vi "Path Edit.vi"() -> ()   [LabVIEW 2013]
uses:
  Global Variables.vi
panel:
  in  "Index":i32=8
  in  "Direction":u16(ring) items=["Forward", "Backward"]
  in  "Enabled":bool=TRUE
  in  "Voltage Schedule":u16(ring) items=["Constant", "Ramp", "Fn. Generator", "Formula"]
  in  "Apply to All":bool
  in  "Fill Orientation":u16(ring) items=["Horizontal", "Vertical"]
  in  "Smooth Segments":dbl=12.0
  in  "Speed Schedule":u16(ring) items=["Constant", "Ramp", "Fn. Generator", "Formula"]
  in  "Speed (µm/s)":dbl=8.0
  in  "Voltage (V)":dbl=8.0
  in  "Speed Settings":bool
  in  "Voltage Settings":bool
  in  "Fill Spacing":dbl=0.1
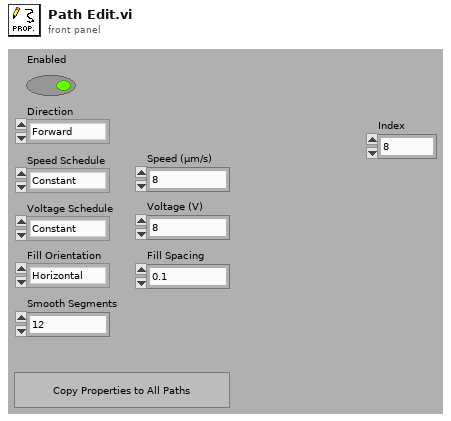
[diagram p1: front panel]
types:
  T1 = enum32{"invalid app kind", "Development System", "Run Time System", "Student Edition", "Embedded LabVIEW", "Evaluation", "Custom"}
  T2 = enum32{"Invalid", "Standard", "Closed", "Hidden", "Minimized", "Maximized"}
  T3 = cluster{"Enabled":bool, "Direction":u16, "Fill Orientation":u16, "Smooth Segments":dbl, "Fill Spacing":dbl, "Speed (µm/s)":cluster{"Schedule":u16, "Value":dbl, "Start Value":dbl, "End Value":dbl, "Min Value":dbl, "Max Value":dbl, "Duty Cycle (%)":dbl, "Signal Type":u16, "Cycle Number":dbl, "Phase (degrees)":dbl}, "Voltage (V)":cluster{"Schedule":u16, "Value":dbl, "Start Value":dbl, "End Value":dbl, "Min Value":dbl, "Max Value":dbl, "Duty Cycle (%)":dbl, "Signal Type":u16, "Cycle Number":dbl, "Phase (degrees)":dbl}}[]
  T4 = cluster{"Enabled":bool, "Direction":u16, "Fill Orientation":u16, "Smooth Segments":dbl, "Fill Spacing":dbl, "Speed (µm/s)":cluster{"Schedule":u16, "Value":dbl, "Start Value":dbl, "End Value":dbl, "Min Value":dbl, "Max Value":dbl, "Duty Cycle (%)":dbl, "Signal Type":u16, "Cycle Number":dbl, "Phase (degrees)":dbl}, "Voltage (V)":cluster{"Schedule":u16, "Value":dbl, "Start Value":dbl, "End Value":dbl, "Min Value":dbl, "Max Value":dbl, "Duty Cycle (%)":dbl, "Signal Type":u16, "Cycle Number":dbl, "Phase (degrees)":dbl}}
  T5 = cluster{"Schedule":u16, "Value":dbl, "Start Value":dbl, "End Value":dbl, "Min Value":dbl, "Max Value":dbl, "Duty Cycle (%)":dbl, "Signal Type":u16, "Cycle Number":dbl, "Phase (degrees)":dbl}
  T6 = cluster{"Schedule":u16, "Value":dbl, "Start Value":dbl, "End Value":dbl, "Min Value":dbl, "Max Value":dbl, "Duty Cycle (%)":dbl, "Speed Signal Type":u16, "Cycle Number":dbl, "Phase (degrees)":dbl}
  T7 = cluster{"Core":cluster{"Current VI Reference":refnum<vi>, "Close Panel on Exit?":bool}}
  T8 = cluster{"Current VI Reference":refnum<vi>, "Close Panel on Exit?":bool}
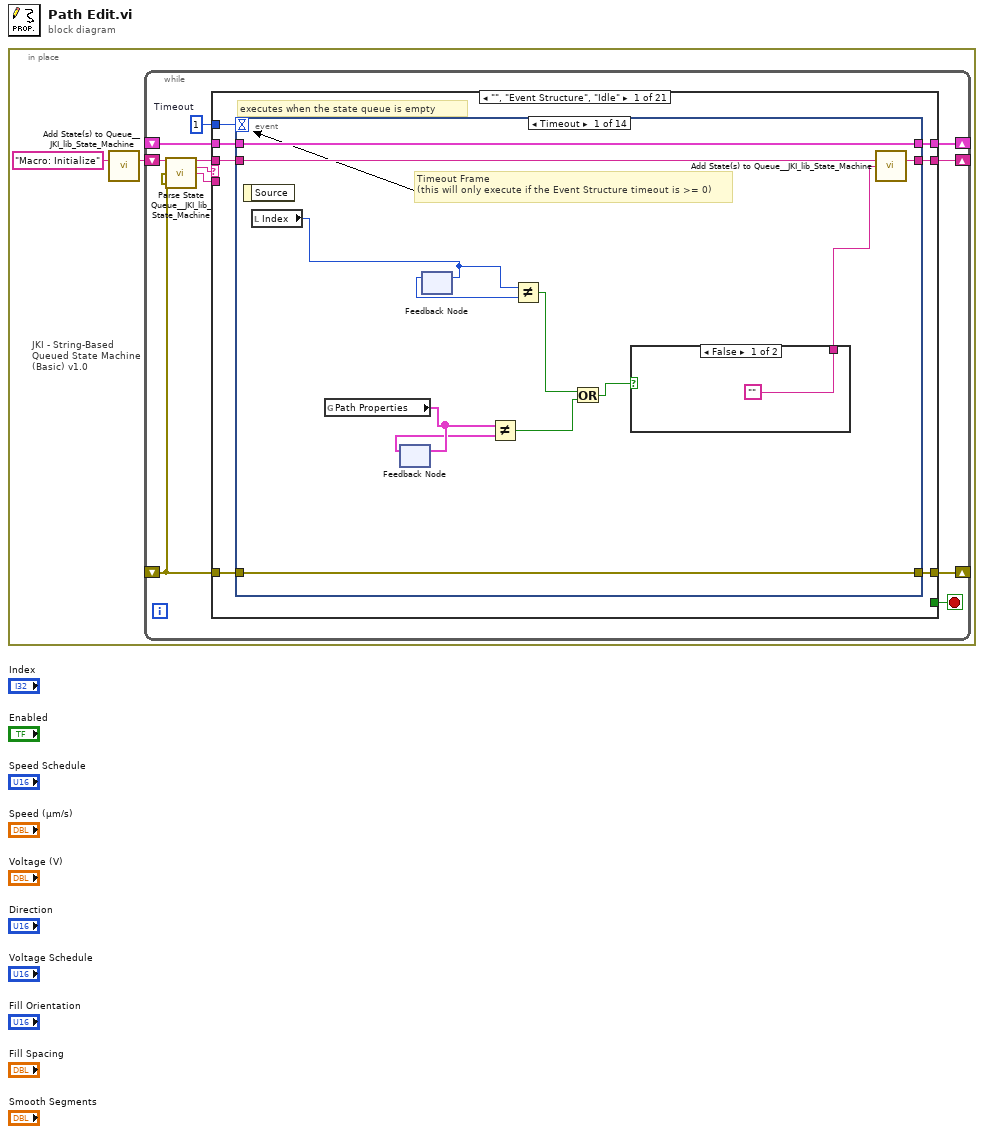
[diagram p0: block diagram]
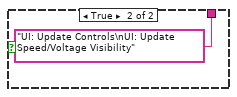
[diagram p2: hidden frame]
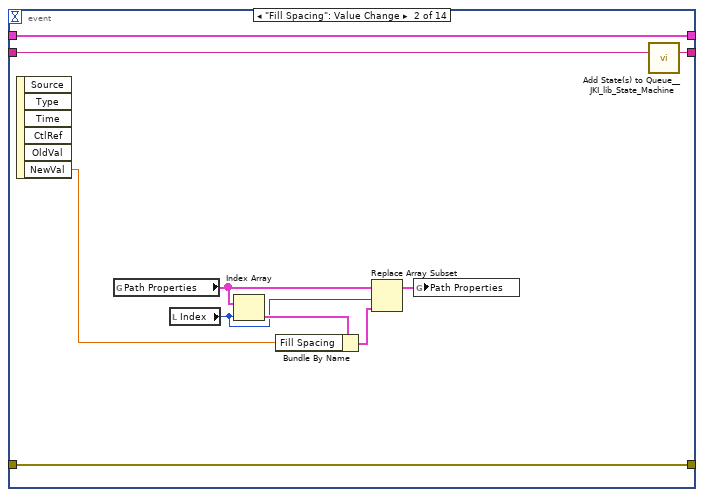
[diagram p3: hidden frame]
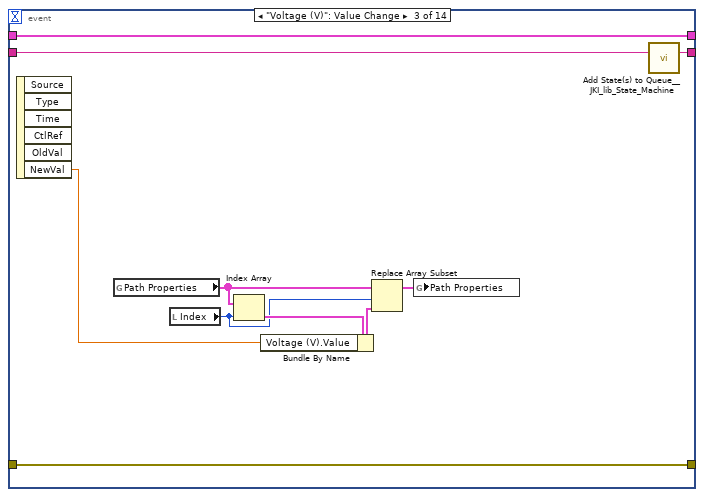
[diagram p4: hidden frame]
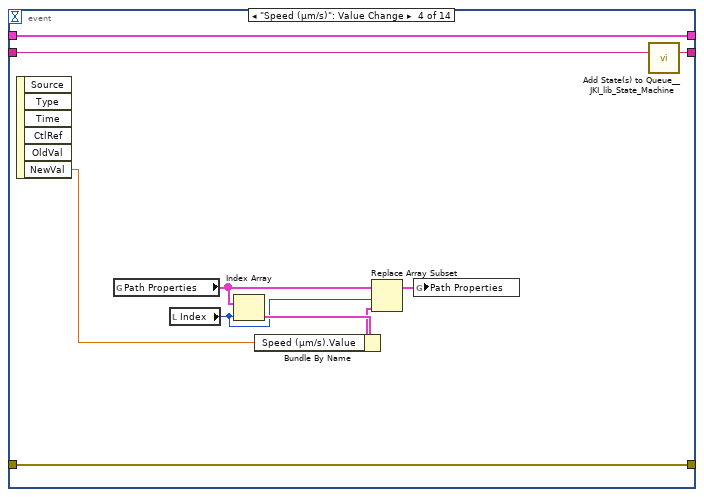
[diagram p5: hidden frame]
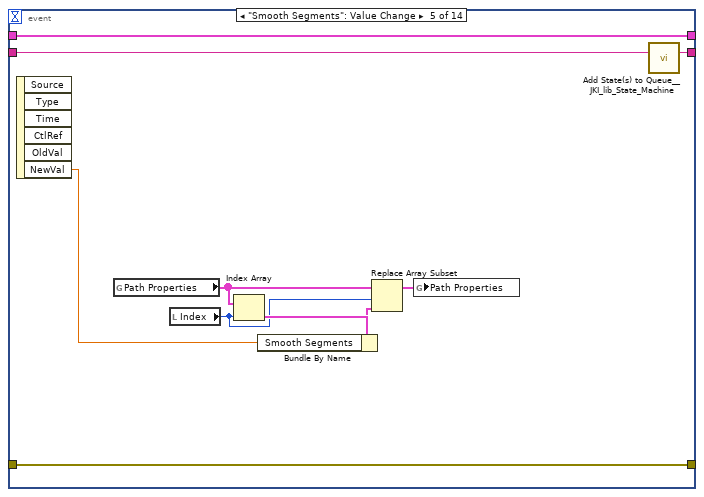
[diagram p6: hidden frame]
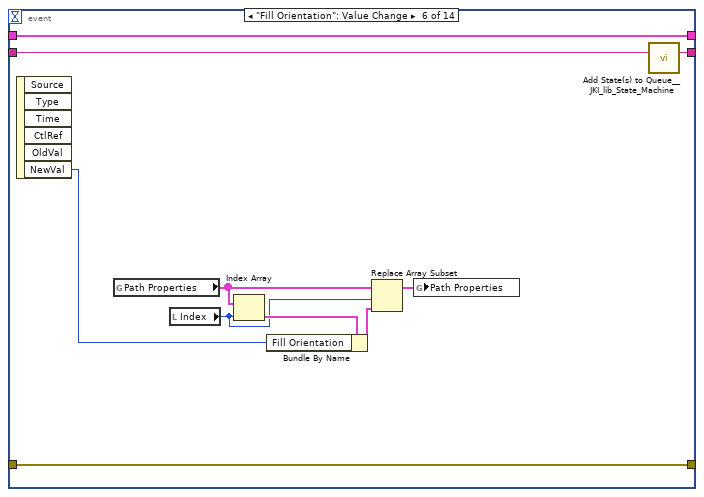
[diagram p7: hidden frame]
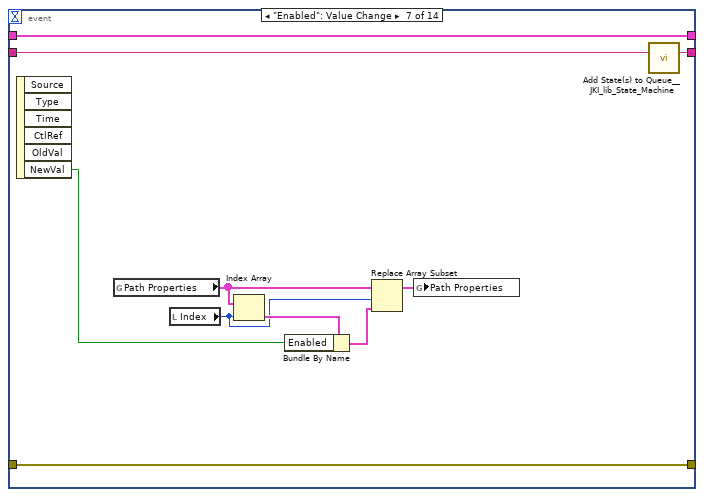
[diagram p8: hidden frame]
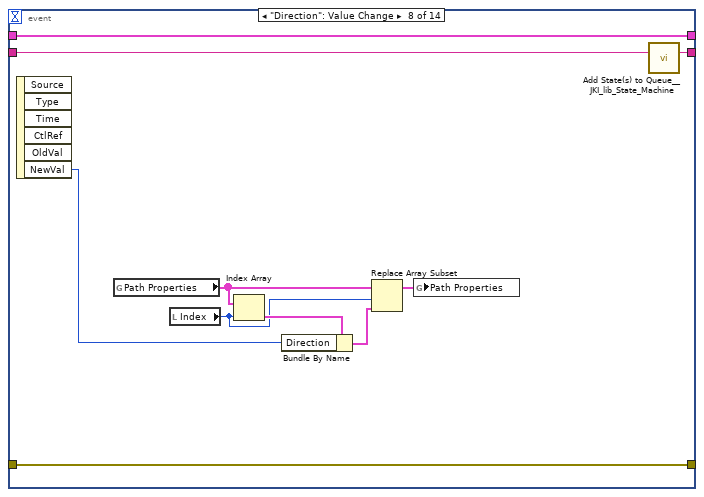
[diagram p9: hidden frame]
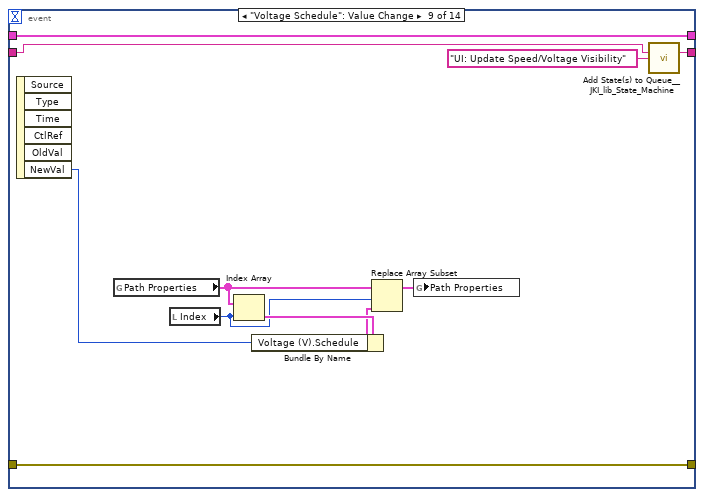
[diagram p10: hidden frame]
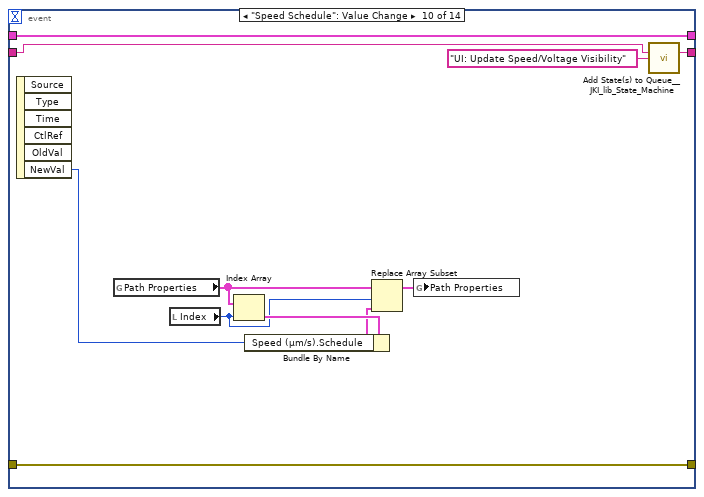
[diagram p11: hidden frame]
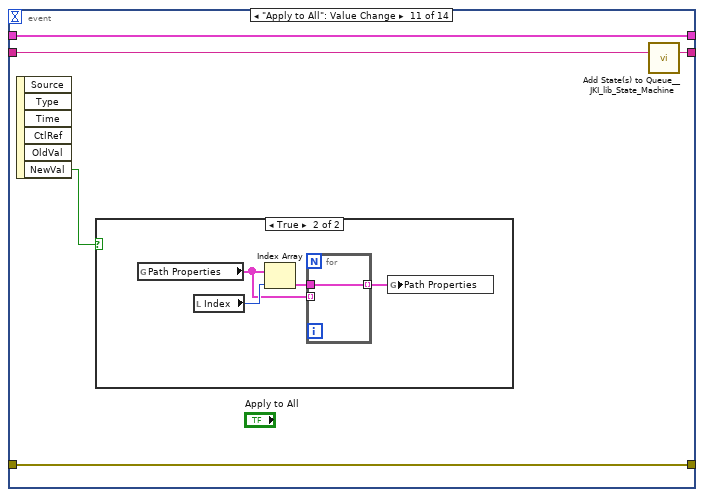
[diagram p12: hidden frame]
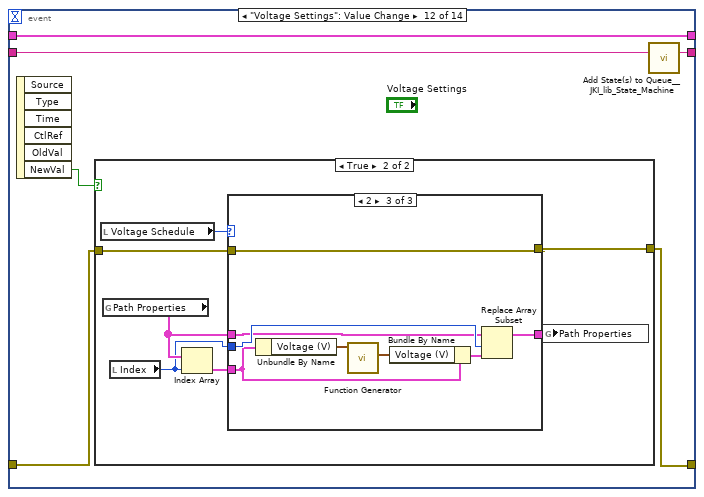
[diagram p14: hidden frame]
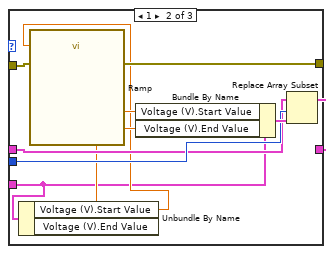
[diagram p17: hidden frame]
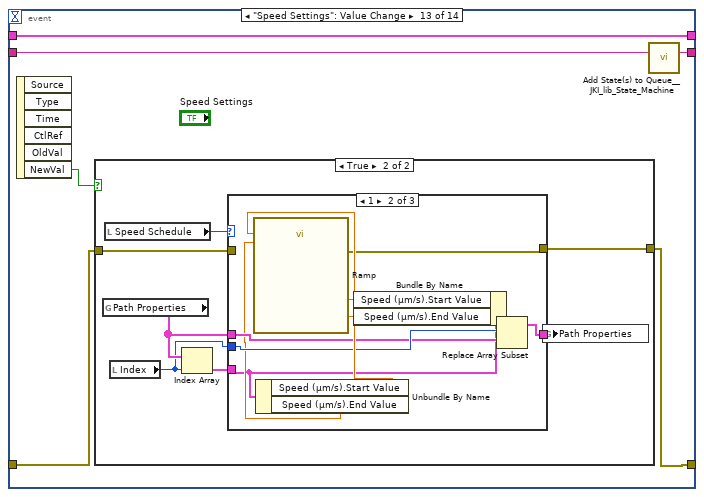
[diagram p18: hidden frame]
diagram:
  n1 = in-place {
    n2 = call <vilib>:"Add State(s) to Queue__JKI_lib_State_Machine.vi"("State(s) in (\"\")"="Macro: Initialize") -> ("States Out"=w2:string)  [unwired: 14 in]
    n3 = while "JKI - String-Based Queued State Machine (Basic) v1.0" {
      shift-right: [w6] -> _
      shift-left: _ -> [w5]
      shift-right: [w9] -> _
      shift-left: _ -> [w3]
      shift-right: [w8] -> _
      shift-left: w2 -> [w10]
      stop <- w7 stop-if-true
      w4 = 1  # Timeout
      n4 = call <vilib>:"Parse State Queue__JKI_lib_State_Machine.vi"("State Queue"=w10, "Error In (no error)"=w3) -> ("Remaining States"=w12:string, "Current State"=w13:string, "Arguments"=w11:string)  [unwired: 11 in]
      n5 = case shown="\"\", \"Event Structure\", \"Idle\"" w13 {
        selector: w13 -> [_ _ w216 _ _ _ _ _ _ _ _ _ _ _ _ _ _ _ _ _ _]
        tunnel: w12 -> [w20 w215 w220 w238 w244 w249 w253 w258 w264 w268 w272 w288 w294 w312 w323 w349 w354 w364 w368 w372 w376]
        tunnel: w11 -> [_ _ _ _ _ _ _ _ _ _ _ _ w289 _ w317 _ _ _ _ _ _]
        tunnel: w5 -> [w18 w212 w218 w234 w241 w247 w250 _ w262 w265 w270 w286 w292 w310 w319 w346 w351 w361 w365 w369 w373]
        tunnel: [w17 w213 w222 w235 errorcluster {"status"=FALSE, "code"=0, "source"=""} ("error out") w246 w251 w254 w260 w266 w269 w285 w290 w299 w320 w347 w352 w362 w366 w370 w374] -> w9
        tunnel: w3 -> [w16 w213 w221 w235 w240 w246 w251 w254 w259 w266 w269 w285 w291 w309 w321 w347 w352 w362 w366 w370 w374]
        tunnel: [w19 w214 w219 w237 w243 w248 w252 w257 w263 w267 w271 w287 w293 w311 w322 w348 w353 w363 w367 w371 w375] -> w8
        tunnel: [_ _ _ _ _ TRUE _ _ _ _ _ _ _ _ _ _ _ _ _ _ _] -> w7
        tunnel: [w15 w212 w218 w236 w241 w247 w250 w256 w262 w265 w270 w286 w292 w310 w319 w346 w351 w361 w365 w369 w373] -> w6
        tunnel: w4 -> [w14 _ _ _ _ _ _ _ _ _ _ _ _ _ _ _ _ _ _ _ _]
        frame "", "Event Structure", "Idle" {
          # "executes when the state queue is empty"
          n6 = event shown="[0] Timeout" {
            selector: _ -> [_ _ _ _ _ _ _ _ _ _ _ _ _ _]
            dyn-events: _ -> [_ _ _ _ _ _ _ _ _ _ _ _ _ _]
            timeout: w14 -> [_ _ _ _ _ _ _ _ _ _ _ _ _ _]
            tunnel: w20 -> [w32 w44 w54 w64 w74 w84 w94 w104 w115 w126 w131 w142 w177 w211]
            tunnel: [w31 w43 w53 w63 w73 w83 w93 w103 w114 w125 w130 w141 w176 w210] -> w19
            tunnel: w18 -> [w29 w42 w52 w62 w72 w82 w92 w102 w113 w124 w129 w140 w175 w208]
            tunnel: [w30 w36 w46 w56 w66 w76 w86 w96 w107 w118 w128 w138 w173 w209] -> w17
            tunnel: w16 -> [w30 w36 w46 w56 w66 w76 w86 w96 w107 w118 w128 w139 w174 w209]
            tunnel: [w29 w42 w52 w62 w72 w82 w92 w102 w113 w124 w129 w140 w175 w208] -> w15
            event Timeout {
              # "Timeout Frame\n(this will only execute if the Event Structure timeout is >= 0)"
              n7 = event-data() -> ()  [unwired: 1 in, 1 out]
              n8 = local read "Index"() -> (w27:i32)
              n9 = global read "Global Variables.vi" "Path Properties"() -> (w26:T3)
              n10 = feedback #1() -> (w25:T3)  [unwired: 1 in]
              n11 = feedback-in #1(w26) -> ()
              n12 = feedback #2() -> (w28:i32)  [unwired: 1 in]
              n13 = feedback-in #2(w27) -> ()
              n14 = Not Equal?(x=w26, y=w25) -> (x != y?=w23:bool)
              n15 = Not Equal?(x=w27, y=w28) -> (x != y?=w24:bool)
              n16 = Or(x=w24, y=w23) -> (x .or. y?=w22:bool)
              n17 = case shown="False" w22 {
                tunnel: ["" "UI: Update Controls\nUI: Update Speed/Voltage Visibility"] -> w21
                frame False {
                }
                frame True {
                }
              }
              n18 = call <vilib>:"Add State(s) to Queue__JKI_lib_State_Machine.vi"("State(s) in (\"\")"=w32, "State(s) at Back (\"\")"=w21) -> ("States Out"=w31:string)  [unwired: 13 in]
            }
            event "Fill Spacing": Value Change {
              n19 = event-data() -> ("NewVal"=w40:dbl)  [unwired: 1 in, 5 out]
              n20 = global read "Global Variables.vi" "Path Properties"() -> (w38:T3)
              n21 = local read "Index"() -> (w35:i32)
              n22 = Index Array(array=w38, index=w35) -> (element=w41:T4)
              n23 = Bundle By Name(cluster=w41, "Fill Spacing"=w40) -> (w39:T4)
              n24 = Replace Array Subset(array=w38, new element=w39, index=w35) -> (w37:T3)
              n25 = global write "Global Variables.vi" "Path Properties"(w37) -> ()
              n26 = call <vilib>:"Add State(s) to Queue__JKI_lib_State_Machine.vi"("State(s) in (\"\")"=w44) -> ("States Out"=w43:string)  [unwired: 14 in]
            }
            event "Voltage (V)": Value Change {
              n27 = event-data() -> ("NewVal"=w50:dbl)  [unwired: 1 in, 5 out]
              n28 = global read "Global Variables.vi" "Path Properties"() -> (w48:T3)
              n29 = local read "Index"() -> (w45:i32)
              n30 = Index Array(array=w48, index=w45) -> (element=w51:T4)
              n31 = Bundle By Name(cluster=w51, "Voltage (V).Value"=w50) -> (w49:T4)
              n32 = Replace Array Subset(array=w48, new element=w49, index=w45) -> (w47:T3)
              n33 = global write "Global Variables.vi" "Path Properties"(w47) -> ()
              n34 = call <vilib>:"Add State(s) to Queue__JKI_lib_State_Machine.vi"("State(s) in (\"\")"=w54) -> ("States Out"=w53:string)  [unwired: 14 in]
            }
            event "Speed (µm/s)": Value Change {
              n35 = event-data() -> ("NewVal"=w60:dbl)  [unwired: 1 in, 5 out]
              n36 = global read "Global Variables.vi" "Path Properties"() -> (w58:T3)
              n37 = local read "Index"() -> (w55:i32)
              n38 = Index Array(array=w58, index=w55) -> (element=w61:T4)
              n39 = Bundle By Name(cluster=w61, "Speed (µm/s).Value"=w60) -> (w59:T4)
              n40 = Replace Array Subset(array=w58, new element=w59, index=w55) -> (w57:T3)
              n41 = global write "Global Variables.vi" "Path Properties"(w57) -> ()
              n42 = call <vilib>:"Add State(s) to Queue__JKI_lib_State_Machine.vi"("State(s) in (\"\")"=w64) -> ("States Out"=w63:string)  [unwired: 14 in]
            }
            event "Smooth Segments": Value Change {
              n43 = event-data() -> ("NewVal"=w70:dbl)  [unwired: 1 in, 5 out]
              n44 = global read "Global Variables.vi" "Path Properties"() -> (w68:T3)
              n45 = local read "Index"() -> (w65:i32)
              n46 = Index Array(array=w68, index=w65) -> (element=w71:T4)
              n47 = Bundle By Name(cluster=w71, "Smooth Segments"=w70) -> (w69:T4)
              n48 = Replace Array Subset(array=w68, new element=w69, index=w65) -> (w67:T3)
              n49 = global write "Global Variables.vi" "Path Properties"(w67) -> ()
              n50 = call <vilib>:"Add State(s) to Queue__JKI_lib_State_Machine.vi"("State(s) in (\"\")"=w74) -> ("States Out"=w73:string)  [unwired: 14 in]
            }
            event "Fill Orientation": Value Change {
              n51 = event-data() -> ("NewVal"=w80:u16)  [unwired: 1 in, 5 out]
              n52 = global read "Global Variables.vi" "Path Properties"() -> (w78:T3)
              n53 = local read "Index"() -> (w75:i32)
              n54 = Index Array(array=w78, index=w75) -> (element=w81:T4)
              n55 = Bundle By Name(cluster=w81, "Fill Orientation"=w80) -> (w79:T4)
              n56 = Replace Array Subset(array=w78, new element=w79, index=w75) -> (w77:T3)
              n57 = global write "Global Variables.vi" "Path Properties"(w77) -> ()
              n58 = call <vilib>:"Add State(s) to Queue__JKI_lib_State_Machine.vi"("State(s) in (\"\")"=w84) -> ("States Out"=w83:string)  [unwired: 14 in]
            }
            event "Enabled": Value Change {
              n59 = event-data() -> ("NewVal"=w90:bool)  [unwired: 1 in, 5 out]
              n60 = global read "Global Variables.vi" "Path Properties"() -> (w88:T3)
              n61 = local read "Index"() -> (w85:i32)
              n62 = Index Array(array=w88, index=w85) -> (element=w91:T4)
              n63 = Bundle By Name(cluster=w91, "Enabled"=w90) -> (w89:T4)
              n64 = Replace Array Subset(array=w88, new element=w89, index=w85) -> (w87:T3)
              n65 = global write "Global Variables.vi" "Path Properties"(w87) -> ()
              n66 = call <vilib>:"Add State(s) to Queue__JKI_lib_State_Machine.vi"("State(s) in (\"\")"=w94) -> ("States Out"=w93:string)  [unwired: 14 in]
            }
            event "Direction": Value Change {
              n67 = event-data() -> ("NewVal"=w100:u16)  [unwired: 1 in, 5 out]
              n68 = global read "Global Variables.vi" "Path Properties"() -> (w98:T3)
              n69 = local read "Index"() -> (w95:i32)
              n70 = Index Array(array=w98, index=w95) -> (element=w101:T4)
              n71 = Bundle By Name(cluster=w101, "Direction"=w100) -> (w99:T4)
              n72 = Replace Array Subset(array=w98, new element=w99, index=w95) -> (w97:T3)
              n73 = global write "Global Variables.vi" "Path Properties"(w97) -> ()
              n74 = call <vilib>:"Add State(s) to Queue__JKI_lib_State_Machine.vi"("State(s) in (\"\")"=w104) -> ("States Out"=w103:string)  [unwired: 14 in]
            }
            event "Voltage Schedule": Value Change {
              n75 = event-data() -> ("NewVal"=w111:u16)  [unwired: 1 in, 5 out]
              n76 = global read "Global Variables.vi" "Path Properties"() -> (w109:T3)
              n77 = local read "Index"() -> (w105:i32)
              n78 = Index Array(array=w109, index=w105) -> (element=w112:T4)
              n79 = Bundle By Name(cluster=w112, "Voltage (V).Schedule"=w111) -> (w110:T4)
              n80 = Replace Array Subset(array=w109, new element=w110, index=w105) -> (w108:T3)
              n81 = global write "Global Variables.vi" "Path Properties"(w108) -> ()
              n82 = call <vilib>:"Add State(s) to Queue__JKI_lib_State_Machine.vi"("State(s) in (\"\")"=w115, "State(s) at Back (\"\")"="UI: Update Speed/Voltage Visibility" ("State(s) at Back (\"\")")) -> ("States Out"=w114:string)  [unwired: 13 in]
            }
            event "Speed Schedule": Value Change {
              n83 = event-data() -> ("NewVal"=w122:u16)  [unwired: 1 in, 5 out]
              n84 = global read "Global Variables.vi" "Path Properties"() -> (w120:T3)
              n85 = local read "Index"() -> (w116:i32)
              n86 = Index Array(array=w120, index=w116) -> (element=w123:T4)
              n87 = Bundle By Name(cluster=w123, "Speed (µm/s).Schedule"=w122) -> (w121:T4)
              n88 = Replace Array Subset(array=w120, new element=w121, index=w116) -> (w119:T3)
              n89 = global write "Global Variables.vi" "Path Properties"(w119) -> ()
              n90 = call <vilib>:"Add State(s) to Queue__JKI_lib_State_Machine.vi"("State(s) in (\"\")"=w126, "State(s) at Back (\"\")"="UI: Update Speed/Voltage Visibility" ("State(s) at Back (\"\")")) -> ("States Out"=w125:string)  [unwired: 13 in]
            }
            event "Apply to All": Value Change {
              n91 = event-data() -> ("NewVal"=w127:bool)  [unwired: 1 in, 5 out]
              n92 = case shown="True" w127 {
                frame False {
                }
                frame True {
                  n93 = global read "Global Variables.vi" "Path Properties"() -> (w132:T3)
                  n94 = local read "Index"() -> (w135:i32)
                  n95 = Index Array(array=w132, index=w135) -> (element=w134:T4)
                  n96 = for {
                    tunnel: w134 -> [w136]
                    tunnel: [w136] -> w133 mode=indexing
                    tunnel: w132 -> [_] mode=indexing
                  }
                  n97 = global write "Global Variables.vi" "Path Properties"(w133) -> ()
                }
              }
              n98 = call <vilib>:"Add State(s) to Queue__JKI_lib_State_Machine.vi"("State(s) in (\"\")"=w131) -> ("States Out"=w130:string)  [unwired: 14 in]
            }
            event "Voltage Settings": Value Change {
              n99 = event-data() -> ("NewVal"=w137:bool)  [unwired: 1 in, 5 out]
              n100 = case shown="True" w137 {
                tunnel: w139 -> [w143 w149]
                tunnel: [w143 w148] -> w138
                frame False {
                }
                frame True {
                  n101 = local read "Voltage Schedule"() -> (w150:u16)
                  n102 = global read "Global Variables.vi" "Path Properties"() -> (w145:T3)
                  n103 = local read "Index"() -> (w144:i32)
                  n104 = Index Array(array=w145, index=w144) -> (element=w146:T4)
                  n105 = case shown="2" w150 {
                    tunnel: w149 -> [w152 w163 w167]
                    tunnel: [w152 w156 w167] -> w148
                    tunnel: [w151 w157 w168] -> w147
                    tunnel: w146 -> [_ w153 w166]
                    tunnel: w145 -> [w151 w158 w169]
                    tunnel: w144 -> [_ w159 w170]
                    frame 0, Default {
                    }
                    frame 1 {
                      n106 = Unbundle By Name(w153) -> ("Voltage (V).Start Value"=w155:dbl, "Voltage (V).End Value"=w154:dbl)
                      n107 = call "Ramp.vi"("Start Value"=w155, "End Value"=w154, "error in (no error)"=w163) -> ("End Value"=w161:dbl, "Start Value"=w162:dbl, "error out"=w156:errorcluster)  [unwired: 13 in, 1 out]
                      n108 = Bundle By Name(cluster=w153, "Voltage (V).Start Value"=w162, "Voltage (V).End Value"=w161) -> (w160:T4)
                      n109 = Replace Array Subset(array=w158, new element=w160, index=w159) -> (w157:T3)
                    }
                    frame 2 {
                      n110 = Unbundle By Name(w166) -> ("Voltage (V)"=w164:T5)
                      n111 = call "Function Generator.vi"("Properties in"=w164) -> ("Properties out"=w165:T6)  [unwired: 9 in, 1 out]
                      n112 = Bundle By Name(cluster=w166, "Voltage (V)"=w165) -> (w171:T4)
                      n113 = Replace Array Subset(array=w169, new element=w171, index=w170) -> (w168:T3)
                    }
                  }
                  n114 = global write "Global Variables.vi" "Path Properties"(w147) -> ()
                }
              }
              n115 = call <vilib>:"Add State(s) to Queue__JKI_lib_State_Machine.vi"("State(s) in (\"\")"=w142) -> ("States Out"=w141:string)  [unwired: 14 in]
            }
            event "Speed Settings": Value Change {
              n116 = event-data() -> ("NewVal"=w172:bool)  [unwired: 1 in, 5 out]
              n117 = case shown="True" w172 {
                tunnel: w174 -> [w178 w184]
                tunnel: [w178 w183] -> w173
                frame False {
                }
                frame True {
                  n118 = global read "Global Variables.vi" "Path Properties"() -> (w180:T3)
                  n119 = local read "Speed Schedule"() -> (w185:u16)
                  n120 = local read "Index"() -> (w179:i32)
                  n121 = Index Array(array=w180, index=w179) -> (element=w181:T4)
                  n122 = case shown="1" w185 {
                    tunnel: w184 -> [w187 _ w201]
                    tunnel: [w187 w193 w201] -> w183
                    tunnel: [w186 w192 w202] -> w182
                    tunnel: w181 -> [_ w188 w200]
                    tunnel: w180 -> [w186 w190 w203]
                    tunnel: w179 -> [_ w191 w204]
                    frame 0, Default {
                    }
                    frame 1 {
                      n123 = Unbundle By Name(w188) -> ("Speed (µm/s).Start Value"=w194:dbl, "Speed (µm/s).End Value"=w189:dbl)
                      n124 = call "Ramp.vi"("Start Value"=w194, "End Value"=w189) -> ("End Value"=w196:dbl, "Start Value"=w197:dbl, "error out"=w193:errorcluster)  [unwired: 14 in, 1 out]
                      n125 = Bundle By Name(cluster=w188, "Speed (µm/s).Start Value"=w197, "Speed (µm/s).End Value"=w196) -> (w195:T4)
                      n126 = Replace Array Subset(array=w190, new element=w195, index=w191) -> (w192:T3)
                    }
                    frame 2 {
                      n127 = Unbundle By Name(w200) -> ("Speed (µm/s)"=w198:T5)
                      n128 = call "Function Generator.vi"("Properties in"=w198) -> ("Properties out"=w199:T6)  [unwired: 9 in, 1 out]
                      n129 = Bundle By Name(cluster=w200, "Speed (µm/s)"=w199) -> (w205:T4)
                      n130 = Replace Array Subset(array=w203, new element=w205, index=w204) -> (w202:T3)
                    }
                  }
                  n131 = global write "Global Variables.vi" "Path Properties"(w182) -> ()
                }
              }
              n132 = call <vilib>:"Add State(s) to Queue__JKI_lib_State_Machine.vi"("State(s) in (\"\")"=w177) -> ("States Out"=w176:string)  [unwired: 14 in]
            }
            event Panel Close? {
              # "Discard the event because we'll close the front panel ourselves in Macro: Exit"
              # "Close Panel button (pressed) Event\n(this executes Macro: Exit to terminate the VI)"
              n133 = event-data() -> ()  [unwired: 1 in, 1 out]
              n134 = event-data("Discard?"=TRUE) -> ()  [unwired: 1 in, 1 out]
              n135 = call <vilib>:"Add State(s) to Queue__JKI_lib_State_Machine.vi"("State(s) in Front (\"\")"="Macro: Exit", "State(s) in (\"\")"=w211) -> ("States Out"=w210:string)  [unwired: 13 in]
            }
          }
        }
        frame "---------- Core ----------" {
          # "Do not put any code in this frame.\n(it is a separator no-op)"
          n136 = call <vilib>:"Add State(s) to Queue__JKI_lib_State_Machine.vi"("State(s) in (\"\")"=w215) -> ("States Out"=w214:string)  [unwired: 14 in]
        }
        frame Default {
          w225 = 42 items=["No error", "Argument error", "Memory is full", "Out of zone", "End of file", "File already open", "Generic file I/O error", "File not found", "File permission error", "Disk is full", "Duplicate path", "Too many files open", "System feature not enabled", "Resource file not found", "Cannot add resource", "Resource not found", "Image not found", "Image memory error", "Pen does not exist", "Config type invalid", "Config token not found", "Config parse error", "Config memory error", "Bad external code format", "Bad external code offset", "External code not present", "Null window", "Destroy window error", "Null menu", "Print aborted", "Bad print record", "Print driver error", "Windows error during printing", "Memory error during printing", "Print dialog error", "Generic print error", "Invalid device refnum", "Device not found", "Device parameter error", "Device unit error", "Cannot open device", "Device call aborted", "Generic error", "Cancelled by user", "Object ID too low", "Object ID too high", "Object not in heap", "Unknown heap", "Unknown object (invalid DefProc)", "Unknown object (DefProc not in table)", "Message out of range", "Invalid (null) method", "Unknown message", "Manager call not supported", "Bad address", "Network operation in progress", "Network operation timed out", "Connection is busy", "Network attribute not supported", "Network error", "Address in use", "System out of memory", "Connection aborted", "Connection refused", "Not connected", "Already connected", "Connection closed", "Initialization error (interapplication manager)", "Bad occurrence", "Wait on unbound occurrence handler", "Occurrence queue overflow", "Datalog type conflict", "Unused", "Unrecognized type (interapplication manager)", "Memory corrupt", "Failed to make temporary DLL", "Old CIN version", "Drag socket not found", "Failed to load drop-object", "Failed to register OLE object", "Failed to release OLE object", "Format specifier type mismatch", "Unknown format specifier", "Too few format specifiers", "Too many format specifiers", "Scan failed", "Newer CIN version", "Error converting to variant", "Runtime menu error", "Password tampered", "Variant attribute not found", "Incompatible variant data type", "Event data is not available", "Event Store is not present", "Occurrence is not found", "Event Queue is not created", "Event info is not available", "Refnum passed is NULL", "Error retrieving Class GUID", "Error retrieving CoClass GUID", "Error retrieving TypeLib GUID.", "Bad built application magic bytes.", "Specific driver is different from the specific driver associated with the Logical Name.", "There is no session opened to the class driver.", "Max Error", "MAX - Error with config objects", "MAX - Error loading configuration", "MAX - Group not supported"]
          # "Current State"
          # "Do not delete, rename, or modify this frame.\n(this is used to capture unhandled states and typos)"
          # "Handle mistyped state name (developer tool)"
          n137 = Format Into String(format string="Software Exception: Unhandled State \"%s\"." ("message"), error in=w221, w216) -> (resulting string=w224:string, error out=w223:errorcluster)  [unwired: 1 in]
          n138 = call <vilib>:"Error Cluster From Error Code.vi"("show call chain? (False)"=TRUE, "error in (no error)"=w223, "error message (\"\")"=w224, "error code (0)"=w225) -> ("error out"=w222:errorcluster)  [unwired: 5 in]
          n139 = call <vilib>:"Add State(s) to Queue__JKI_lib_State_Machine.vi"("State(s) in (\"\")"=w220) -> ("States Out"=w219:string)  [unwired: 14 in]
        }
        frame "Initialize Core Data" {
          # "exe?"
          # "If panel starts closed or is an EXE, then close it when we exit"
          # "Do not delete, rename, or modify this frame.\n(this is used to determine panel behavior on exit)"
          n140 = control-ref of="Current VI Reference"() -> (w233:refnum<vi>)
          n141 = property class="VI"() -> ("Front Panel.Open"=w232:bool)  [unwired: 2 in, 2 out]
          n142 = property class="App"() -> ("App.Kind"=w231:T1)  [unwired: 2 in, 2 out]
          n143 = Not(x=w232) -> (.not. x?=w229:bool)
          n144 = Equal?(x=w231, y=T1."Run Time System" ("Application:Kind")) -> (x = y?=w228:bool)
          n145 = Or(x=w229, y=w228) -> (x .or. y?=w227:bool)
          n146 = Bundle By Name(cluster=w234, "Core.Current VI Reference"=w233, "Core.Close Panel on Exit?"=w227) -> (w236:T7)
          n147 = call <vilib>:"Add State(s) to Queue__JKI_lib_State_Machine.vi"("State(s) in (\"\")"=w238) -> ("States Out"=w237:string)  [unwired: 14 in]
        }
        frame "Error Handler" {
          # "Unhandled Error -- Display it"
          # "Handle any errors here.\nYou can also output any states to clean-up after errors occur"
          # "Clear error"
          n148 = call <vilib>:"General Error Handler.vi"("error in (no error)"=w240) -> ()  [unwired: 10 in, 5 out]
          n149 = call <vilib>:"Add State(s) to Queue__JKI_lib_State_Machine.vi"("State(s) in Front (\"\")"="/* Post Error States", "State(s) in (\"\")"=w244) -> ("States Out"=w243:string)  [unwired: 13 in]
        }
        frame "Exit" {
          # "Do not put any code in this frame.\n(No errors that occur here will be handled.)"
          n150 = call <vilib>:"Add State(s) to Queue__JKI_lib_State_Machine.vi"("State(s) in (\"\")"=w249) -> ("States Out"=w248:string)  [unwired: 14 in]
        }
        frame "---------- Data ----------" {
          # "Do not put any code in this frame.\n(It is a separator no-op. You can make a copy of this frame to create a new Data frame)"
          n151 = call <vilib>:"Add State(s) to Queue__JKI_lib_State_Machine.vi"("State(s) in (\"\")"=w253) -> ("States Out"=w252:string)  [unwired: 14 in]
        }
        frame "Data: Initialize" {
          w255 = T8 {"Current VI Reference"=refnum, "Close Panel on Exit?"=FALSE}  # Core
          # "Initialize the shift-register data, here.\n(data names are defined by what you wire into the bundle function)"
          n152 = Bundle("Core"=w255) -> (w256:T7)  [unwired: 1 in]
          n153 = call <vilib>:"Add State(s) to Queue__JKI_lib_State_Machine.vi"("State(s) in (\"\")"=w258) -> ("States Out"=w257:string)  [unwired: 14 in]
        }
        frame "Data: Cleanup" {
          # "Cleanup any data and references, here.\n(this is called automatically, by the Macro: Exit)"
          n154 = Unbundle By Name(w262) -> ("Core.Current VI Reference"=w261:refnum<vi>)
          n155 = Close Reference(reference=w261, error in (no error)=w259) -> (error out=w260:errorcluster)
          n156 = call <vilib>:"Add State(s) to Queue__JKI_lib_State_Machine.vi"("State(s) in (\"\")"=w264) -> ("States Out"=w263:string)  [unwired: 14 in]
        }
        frame "---------- UI ----------" {
          # "Do not put any code in this frame.\n(It is a separator no-op. You can make a copy of this frame to create a new UI frame)"
          n157 = call <vilib>:"Add State(s) to Queue__JKI_lib_State_Machine.vi"("State(s) in (\"\")"=w268) -> ("States Out"=w267:string)  [unwired: 14 in]
        }
        frame "UI: Initialize" {
          # "Initialize the User Interface, here.\n(this is called automatically, by the Macro: Init)"
          n158 = call <vilib>:"Add State(s) to Queue__JKI_lib_State_Machine.vi"("State(s) in (\"\")"=w272) -> ("States Out"=w271:string)  [unwired: 14 in]
        }
        frame "UI: Update Controls" {
          n159 = global read "Global Variables.vi" "Path Properties"() -> (w273:T3)
          n160 = local read "Index"() -> (w277:i32)
          n161 = Index Array(array=w273, index=w277) -> (element=w276:T4)
          n162 = Unbundle By Name(w276) -> ("Enabled"=w278:bool, "Direction"=w279:u16, "Fill Orientation"=w280:u16, "Smooth Segments"=w281:dbl, "Fill Spacing"=w282:dbl, "Speed (µm/s).Schedule"=w275:u16, "Speed (µm/s).Value"=w283:dbl, "Voltage (V).Schedule"=w274:u16, "Voltage (V).Value"=w284:dbl)
          n163 = local write "Enabled"(w278) -> ()
          n164 = local write "Direction"(w279) -> ()
          n165 = local write "Fill Orientation"(w280) -> ()
          n166 = local write "Smooth Segments"(w281) -> ()
          n167 = local write "Fill Spacing"(w282) -> ()
          n168 = local write "Speed Schedule"(w275) -> ()
          n169 = local write "Speed (µm/s)"(w283) -> ()
          n170 = local write "Voltage Schedule"(w274) -> ()
          n171 = local write "Voltage (V)"(w284) -> ()
          n172 = call <vilib>:"Add State(s) to Queue__JKI_lib_State_Machine.vi"("State(s) in (\"\")"=w288) -> ("States Out"=w287:string)  [unwired: 14 in]
        }
        frame "UI: Cursor Set" {
          # "Argument"
          # "Set and Unset Cursor Busy.\n(Usage: \"UI: Cursor Set >> Busy|Idle\")"
          n173 = case shown="\"Idle\", Default" w289 {
            tunnel: w291 -> [w296 w298]
            tunnel: [w295 w297] -> w290
            frame "Idle", Default {
              n174 = call <vilib>:"Unset Busy.vi"("error in (no error)"=w296) -> ("error out"=w295:errorcluster)  [unwired: 10 in]
            }
            frame "Busy" {
              n175 = call <vilib>:"Set Busy.vi"("error in (no error)"=w298) -> ("error out"=w297:errorcluster)  [unwired: 9 in, 1 out]
            }
          }
          n176 = call <vilib>:"Add State(s) to Queue__JKI_lib_State_Machine.vi"("State(s) in (\"\")"=w294) -> ("States Out"=w293:string)  [unwired: 14 in]
        }
        frame "UI: Update Speed/Voltage Visibility" {
          n177 = local read "Voltage Schedule"() -> (w308:u16)
          n178 = case shown="0" w308 {
            tunnel: [TRUE FALSE] -> w304
            frame 0 {
            }
            frame 1, Default {
            }
          }
          n179 = local read "Speed Schedule"() -> (w307:u16)
          n180 = property on="Voltage (V)" class="DigNum (strict)"(error in=w309, "Visible"=w304) -> (error out=w305:errorcluster)  [unwired: 1 in, 1 out]
          n181 = case shown="0" w307 {
            tunnel: [TRUE FALSE] -> w300
            frame 0 {
            }
            frame 1, Default {
            }
          }
          n182 = Not(x=w304) -> (.not. x?=w303:bool)
          n183 = property on="Voltage Settings" class="Bool"(error in=w305, "Visible"=w303) -> (error out=w302:errorcluster)  [unwired: 1 in, 1 out]
          n184 = property on="Speed (µm/s)" class="DigNum (strict)"(error in=w302, "Visible"=w300) -> (error out=w301:errorcluster)  [unwired: 1 in, 1 out]
          n185 = Not(x=w300) -> (.not. x?=w306:bool)
          n186 = property on="Speed Settings" class="Bool"(error in=w301, "Visible"=w306) -> (error out=w299:errorcluster)  [unwired: 1 in, 1 out]
          n187 = call <vilib>:"Add State(s) to Queue__JKI_lib_State_Machine.vi"("State(s) in (\"\")"=w312) -> ("States Out"=w311:string)  [unwired: 14 in]
        }
        frame "UI: Front Panel State" {
          # "Argument"
          # "Set Front Panel Open or Closed\n(Usage: \"UI: Front Panel State >> Open|Close\")"
          n188 = Unbundle By Name(w319) -> ("Core.Current VI Reference"=w318:refnum<vi>)
          n189 = case shown="\"Open\", Default" w317 {
            tunnel: w321 -> [w327 w340]
            tunnel: [w329 w341] -> w320
            tunnel: w318 -> [w328 w338]
            frame "Open", Default {
              n190 = property class="VI"(reference=w328, error in=w327) -> (reference out=w325:refnum<vi>, error out=w326:errorcluster, "Front Panel.Open"=w324:bool)
              n191 = case shown="False" w324 {
                tunnel: [w332 w335] -> w329
                tunnel: w326 -> [w331 w335]
                tunnel: w325 -> [w330 _]
                frame False {
                  n192 = invoke class="VI" method="FP.Open"(reference=w330, error in=w331, "Activate"=TRUE, "State"=T2."Standard") -> (error out=w332:errorcluster)  [unwired: 1 in, 4 out]
                }
                frame True {
                }
              }
            }
            frame "Close" {
              n193 = property class="VI"(reference=w338, error in=w340) -> (reference out=w337:refnum<vi>, error out=w339:errorcluster, "Front Panel.Open"=w336:bool)
              n194 = case shown="True" w336 {
                tunnel: [w342 w345] -> w341
                tunnel: w339 -> [w342 w344]
                tunnel: w337 -> [_ w343]
                frame False {
                }
                frame True {
                  n195 = invoke class="VI" method="FP.Close"(reference=w343, error in=w344) -> (error out=w345:errorcluster)  [unwired: 1 in, 2 out]
                }
              }
            }
          }
          n196 = call <vilib>:"Add State(s) to Queue__JKI_lib_State_Machine.vi"("State(s) in (\"\")"=w323) -> ("States Out"=w322:string)  [unwired: 14 in]
        }
        frame "---------- Macro ----------" {
          # "Do not put any code in this frame.\n(It is a separator no-op. You can make a copy of this frame to create a new Macro frame)"
          n197 = call <vilib>:"Add State(s) to Queue__JKI_lib_State_Machine.vi"("State(s) in (\"\")"=w349) -> ("States Out"=w348:string)  [unwired: 14 in]
        }
        frame "Macro: Initialize" {
          w350 = "Data: Initialize\nInitialize Core Data\nUI: Initialize\nUI: Update Controls\nUI: Update Speed/Voltage Visibility\nUI: Front Panel State >> Close"  # Data: Initialize Initialize Core Data UI: Initialize UI: Update Controls UI: Update Speed/Voltage Visibility UI: Front Panel State >> Close
          # "Initialization Macro\n(This is called once, when the VI starts)"
          n198 = call <vilib>:"Add State(s) to Queue__JKI_lib_State_Machine.vi"("State(s) in Front (\"\")"=w350, "State(s) in (\"\")"=w354) -> ("States Out"=w353:string)  [unwired: 13 in]
        }
        frame "Macro: Exit" {
          # "Exit Macro\n(This is called once, when the VI exits)"
          n199 = Unbundle By Name(w361) -> ("Core.Close Panel on Exit?"=w360:bool)
          n200 = Select(t="UI: Front Panel State >> Close", s=w360, f="") -> (s? t:f=w357:string)
          n201 = call <vilib>:"Add State(s) to Queue__JKI_lib_State_Machine.vi"("State(s) in (\"\")"=w357, "State(s) at Back (\"\")"="Data: Cleanup\nExit") -> ("States Out"=w355:string)  [unwired: 13 in]
          n202 = call <vilib>:"Add State(s) to Queue__JKI_lib_State_Machine.vi"("State(s) in Front (\"\")"=w355, "State(s) in (\"\")"=w364) -> ("States Out"=w363:string)  [unwired: 13 in]
        }
        frame "---------- New Category ----------" {
          # "Template Separator\n(You can make a copy of, or modify, this frame)"
          n203 = call <vilib>:"Add State(s) to Queue__JKI_lib_State_Machine.vi"("State(s) in (\"\")"=w368) -> ("States Out"=w367:string)  [unwired: 14 in]
        }
        frame "New Category: 1" {
          # "Your code here.\n(You can make a copy of, or modify, this frame)"
          n204 = call <vilib>:"Add State(s) to Queue__JKI_lib_State_Machine.vi"("State(s) in (\"\")"=w372) -> ("States Out"=w371:string)  [unwired: 14 in]
        }
        frame "New Category: 2" {
          # "Your code here.\n(You can make a copy of, or modify, this frame)"
          n205 = call <vilib>:"Add State(s) to Queue__JKI_lib_State_Machine.vi"("State(s) in (\"\")"=w376) -> ("States Out"=w375:string)  [unwired: 14 in]
        }
      }
    }
  }
